vi "LED Ctlr Sys Cal Factor DPLM.vi"() -> ()   [LabVIEW 2010]
uses:
  <vilib>/Analysis/NI_AALPro.lvlib
panel:
  in  "LM Rd Dly":u32
  in  "# LEDs":u8=15
  out "Illum (Dst)":dbl format="%#_4g"
  in  "Dst Det":enum16{"Chn1", "Chn2"}(ring)=enum."Chn2"
  in  "Src Det":enum16{"Chn1", "Chn2"}(ring)
  out "error out":errorcluster
  out "Cal Factor":dbl
  out "Current Step":u16
  out "Max Illum LG":dbl caption="Gain_e" format="%.2f"
  out "Cal Factor LG":dbl caption="Gain_e" format="%.5g"
  out "Cal Factor HG":dbl caption="Gain_e" format="%.5g"
  out "Max Illum HG":dbl caption="Gain_e" format="%.2f"
  out "Calibration LG":cluster{dbl[], dbl[]}(graph)
  out "Calibration HG":cluster{dbl[], dbl[]}(graph)
  in  "OK":bool
  out "Status":string
  out "LG Dst Array":dbl[](array[numeric])
  out "HG Dst Array":dbl[](array[numeric])
  out "LG Src Array":dbl[](array[numeric])
  out "HG Src Array":dbl[](array[numeric])
  out "Inten % (Desired)":dbl
  out "Illum (Src)":dbl format="%#_4g"
  in  "DAC Higher Limit":u32=5500
  in  "DAC Lower Limit":u32=300
  in  "Number of Steps":u32=21
  in  "Wavelength":string="1550"
  in  "LED Driver Com Port":refnum<visa-resource-name>="COM9"
  in  "Light Meter Port":refnum<visa-resource-name>="COM5"
  in  "error in (no error)":errorcluster
  # "Ver 1"
  # "Cal Factor Generator (LEDAD)"
  # "ms"
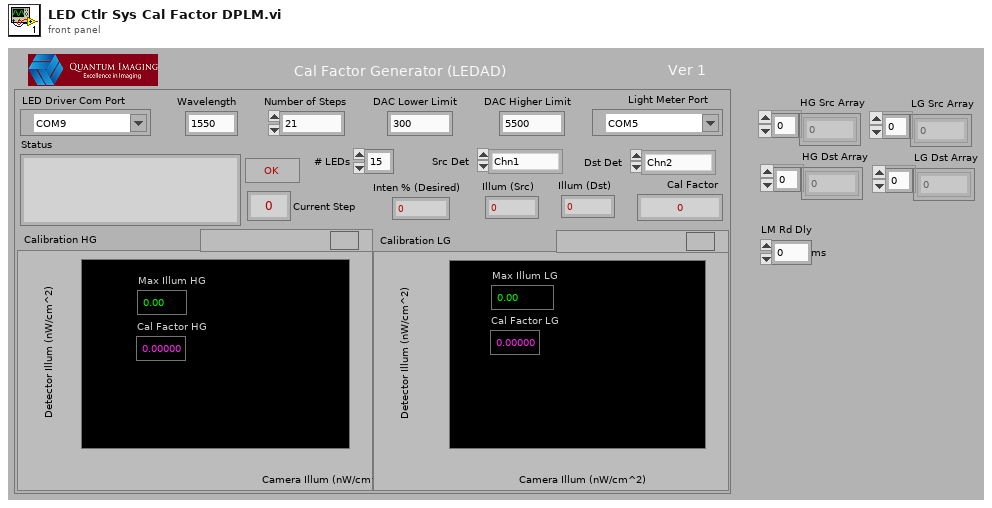
[diagram p1: front panel]
types:
  T1 = cluster{"HG Dst Array":dbl[], "HG Src Array":dbl[]}
  T2 = cluster{"LG Dst Array":dbl[], "LG Src Array":dbl[]}
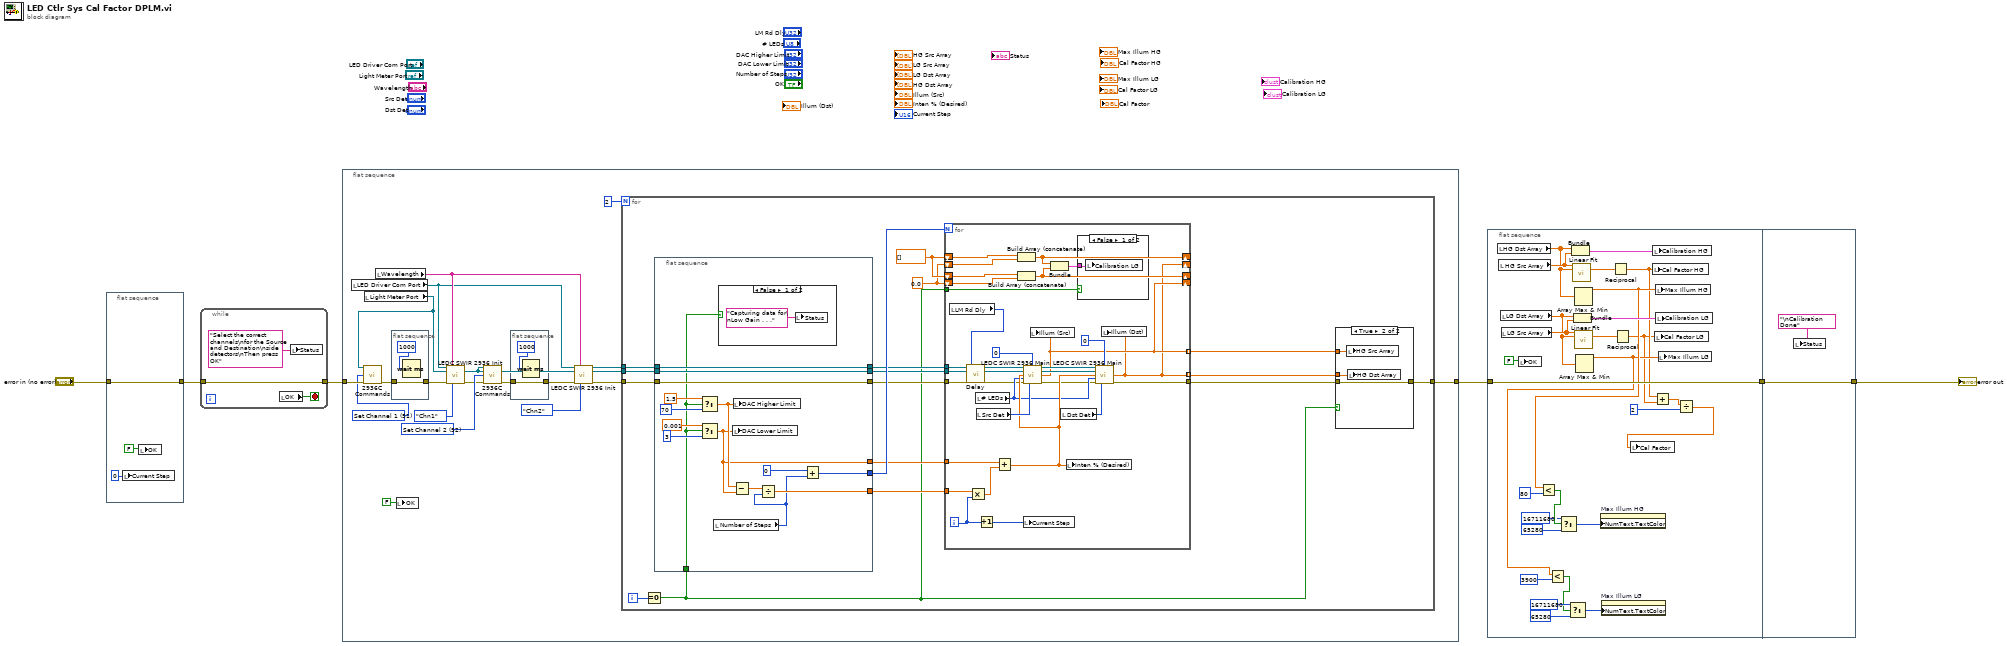
[diagram p0: block diagram]
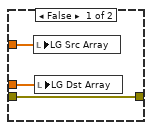
[diagram p2: hidden frame]
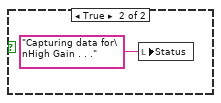
[diagram p3: hidden frame]
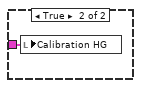
[diagram p4: hidden frame]
diagram:
  n1 = flat-sequence {
    tunnel: "error in (no error)" -> [w7]
    tunnel: [w7] -> w5
    frame #0 {
      n2 = local write "Current Step"(0) -> ()
      n3 = local write "OK"(FALSE) -> ()
    }
  }
  n4 = while {
    tunnel: [w12] -> w4
    tunnel: w5 -> [w12]
    stop <- w10 stop-if-true
    n5 = local read "OK"() -> (w10:bool)
    n6 = local write "Status"("Select the correct channels\nfor the Source and Destination\nside detectors\nThen press OK") -> ()
  }
  n7 = flat-sequence {
    tunnel: w4 -> [w25]
    tunnel: [w32] -> w3
    frame #0 {
      w18 = u16 52 items=["Attenuator OFF", "Attenuator ON", "Attenuator Query", "Beep OFF", "Beep ON", "Beep Query", "Clear Status Reg", "Get Power (nW)", "Echo OFF", "Echo ON", "Echo Query", "No Filter", "Analog Filter", "Digital FIlter", "Filter Query", "Hold", "Go", "Go Query", "Backlight OFF", "Backlight Medium", "Backlight High", "Backlight Query", "Set Dsplay Screen 0", "Set Display Screen 1", "Display Screen Query", "Mode DC Continuous", "Mode DC Single", "Mode Integrate", "Identification", "Auto Range", "Auto Range Query", "Signal Range 0", "Signal Range 1", "Signal Range 2", "Signal Range 3", "Signal Range 4", "Signal Range 5", "Signal Range 6", "Signal Range Query", "Store Reference", "Units W", "Units W/cm2", "Units dBm", "Units Joules", "Units Query", "Set Wavelength", "Wavelength Querry", "Mode Pesk-to-Peak Cont.", "Mode Peak-to-Peak Sing.", "Mode Query", "Channel Querry", "Set Channel 1", "Set Channel 2"] ("Command")
      w22 = u16 51 items=["Attenuator OFF", "Attenuator ON", "Attenuator Query", "Beep OFF", "Beep ON", "Beep Query", "Clear Status Reg", "Get Power (nW)", "Echo OFF", "Echo ON", "Echo Query", "No Filter", "Analog Filter", "Digital FIlter", "Filter Query", "Hold", "Go", "Go Query", "Backlight OFF", "Backlight Medium", "Backlight High", "Backlight Query", "Set Dsplay Screen 0", "Set Display Screen 1", "Display Screen Query", "Mode DC Continuous", "Mode DC Single", "Mode Integrate", "Identification", "Auto Range", "Auto Range Query", "Signal Range 0", "Signal Range 1", "Signal Range 2", "Signal Range 3", "Signal Range 4", "Signal Range 5", "Signal Range 6", "Signal Range Query", "Store Reference", "Units W", "Units W/cm2", "Units dBm", "Units Joules", "Units Query", "Set Wavelength", "Wavelength Querry", "Mode Pesk-to-Peak Cont.", "Mode Peak-to-Peak Sing.", "Mode Query", "Channel Querry", "Set Channel 1", "Set Channel 2"] ("Command")
      n8 = local read "LED Driver Com Port"() -> (w15:refnum<visa-resource-name>)
      n9 = local read "Light Meter Port"() -> (w23:refnum<visa-resource-name>)
      n10 = call "2936C Commands.vi"("Instrument Resource Name"=w23, "Command"=w22, "error in (no error)"=w25) -> ("error out"=w24:errorcluster)  [unwired: 8 in, 4 out]
      n11 = local read "Wavelength"() -> (w29:string)
      n12 = flat-sequence {
        tunnel: [w36] -> w20
        tunnel: w24 -> [w36]
        frame #0 {
          n13 = Wait (ms)(milliseconds to wait=1000) -> ()  [unwired: 1 out]
        }
      }
      n14 = local write "OK"(FALSE) -> ()
      n15 = call "LEDC SWIR 2936 Init.vi"("LEDAD Port"=w15, "Wavelength"=w29, "Light Meter Port"=w23, "error in (no error)"=w20, "Channel"=enum16{"Chn1", "Chn2"}."Chn1") -> ("Light Meter Port out"=w19:refnum<visa-resource-name>, "error out"=w17:errorcluster)  [unwired: 6 in, 3 out]
      n16 = call "2936C Commands.vi"("Instrument Resource Name"=w19, "Command"=w18, "error in (no error)"=w17) -> ("error out"=w13:errorcluster)  [unwired: 8 in, 4 out]
      n17 = flat-sequence {
        tunnel: [w34] -> w16
        tunnel: w13 -> [w34]
        frame #0 {
          n18 = Wait (ms)(milliseconds to wait=1000) -> ()  [unwired: 1 out]
        }
      }
      n19 = call "LEDC SWIR 2936 Init.vi"("LEDAD Port"=w15, "Wavelength"=w29, "Light Meter Port"=w19, "error in (no error)"=w16, "Channel"=enum16{"Chn1", "Chn2"}."Chn2") -> ("LEDAD Port out"=w28:refnum<visa-resource-name>, "Light Meter Port out"=w27:refnum<visa-resource-name>, "error out"=w26:errorcluster)  [unwired: 6 in, 2 out]
      n20 = for {
        N: 2 -> [_]
        tunnel: w28 -> [w48]
        tunnel: w27 -> [w47]
        tunnel: w26 -> [w46]
        tunnel: [w41] -> w32
        i -> [w52]
        w37 = 0.0
        w38 = dbl[] []
        n21 = Equal To 0?(x=w52) -> (x = 0?=w39:bool)
        n22 = flat-sequence {
          tunnel: w39 -> [w62]
          tunnel: [w67] -> w51
          tunnel: [w66] -> w50
          tunnel: [w61] -> w49
          tunnel: [w65] -> w45
          tunnel: w48 -> [w65]
          tunnel: [w64] -> w44
          tunnel: w47 -> [w64]
          tunnel: [w63] -> w43
          tunnel: w46 -> [w63]
          frame #0 {
            n23 = Select(t=1.5, s=w62, f=70) -> (s? t:f=w68:dbl)
            n24 = Select(t=0.001, s=w62, f=3) -> (s? t:f=w66:dbl)
            n25 = local read "Number of Steps"() -> (w60:u32)
            n26 = case shown="False" w62 {
              frame False {
                n27 = local write "Status"("Capturing data for\nLow Gain . . .") -> ()
              }
              frame True {
                n28 = local write "Status"("Capturing data for\nHigh Gain . . .") -> ()
              }
            }
            n29 = local write "DAC Lower Limit"(w66) -> ()
            n30 = local write "DAC Higher Limit"(w68) -> ()
            n31 = Subtract(x=w68, y=w66) -> (x-y=w73:dbl)
            n32 = Divide(x=w73, y=w60) -> (x/y=w61:dbl)
            n33 = Add(x=0, y=w60) -> (x+y=w67:u32)
          }
        }
        n34 = for {
          N: w51 -> [_]
          tunnel: w45 -> [w106]
          tunnel: w44 -> [w105]
          tunnel: w43 -> [w79]
          tunnel: w49 -> [w103]
          tunnel: w50 -> [w101]
          tunnel: [w84] -> w53 mode=indexing
          tunnel: [w81] -> w42
          tunnel: [w83] -> w40 mode=indexing
          shift-right: [w92] -> _
          shift-left: w38 -> [w91]
          shift-right: [w83] -> _
          shift-left: w37 -> [w90]
          shift-right: [w87] -> _
          shift-left: w38 -> [w89]
          shift-right: [w84] -> _
          shift-left: w37 -> [w88]
          tunnel: w39 -> [w86]
          i -> [w100]
          n35 = local read "LM Rd Dly"() -> (w77:u32)
          n36 = call "Delay.vi"("error in (no error)"=w79, "Delay"=w77) -> ("error out"=w78:errorcluster)  [unwired: 17 in]
          n37 = Multiply(x=w103, y=w100) -> (x*y=w102:dbl)
          n38 = local read "# LEDs"() -> (w82:u8)
          n39 = local read "Src Det"() -> (w94:enum16{"Chn1", "Chn2"})
          n40 = Increment(x=w100) -> (x+1=w99:i32)
          n41 = Add(x=w101, y=w102) -> (x+y=w93:dbl)
          n42 = Build Array (concatenate)(w91, w90) -> (w92:dbl[])
          n43 = Build Array (concatenate)(w89, w88) -> (w87:dbl[])
          n44 = call "LEDC SWIR 2936 Main.vi"("LEDAD Port"=w106, "Unit"=0, "Light Meter Port"=w105, "Intensity Desired"=w93, "Enable LED"=w82, "error in (no error)"=w78, "Channel"=w94) -> ("LEDAD Port out"=w97:refnum<visa-resource-name>, "Light Meter Port out"=w96:refnum<visa-resource-name>, "Meas Illum"=w84:dbl, "error out"=w80:errorcluster)  [unwired: 3 in, 2 out]
          n45 = local write "Current Step"(w99) -> ()
          n46 = local write "Illum (Src)"(w84) -> ()
          n47 = Bundle(w92, w87) -> (w85:cluster{dbl[], dbl[]})  [unwired: 1 in]
          n48 = local read "Dst Det"() -> (w95:enum16{"Chn1", "Chn2"})
          n49 = local write "Inten % (Desired)"(w93) -> ()
          n50 = case shown="False" w86 {
            tunnel: w85 -> [w107 w108]
            frame False {
              n51 = local write "Calibration LG"(w107) -> ()
            }
            frame True {
              n52 = local write "Calibration HG"(w108) -> ()
            }
          }
          n53 = call "LEDC SWIR 2936 Main.vi"("LEDAD Port"=w97, "Unit"=0, "Light Meter Port"=w96, "Intensity Desired"=w93, "Enable LED"=w82, "error in (no error)"=w80, "Channel"=w95) -> ("Meas Illum"=w83:dbl, "error out"=w81:errorcluster)  [unwired: 3 in, 4 out]
          n54 = local write "Illum (Dst)"(w83) -> ()
        }
        n55 = case shown="True" w39 {
          tunnel: w53 -> [w56 w59]
          tunnel: [w55 w58] -> w41
          tunnel: w42 -> [w55 w58]
          tunnel: w40 -> [w54 w57]
          frame False {
            n56 = local write "LG Src Array"(w56) -> ()
            n57 = local write "LG Dst Array"(w54) -> ()
          }
          frame True {
            n58 = local write "HG Src Array"(w59) -> ()
            n59 = local write "HG Dst Array"(w57) -> ()
          }
        }
      }
    }
  }
  n60 = flat-sequence {
    tunnel: w3 -> [w129]
    tunnel: [w129] -> w1
    tunnel: [w137] -> w2
    tunnel: w1 -> [w137]
    frame #0 {
      n61 = local read "HG Dst Array"() -> (w127:dbl[])
      n62 = local read "HG Src Array"() -> (w135:dbl[])
      n63 = local read "LG Dst Array"() -> (w126:dbl[])
      n64 = local read "LG Src Array"() -> (w132:dbl[])
      n65 = local write "OK"(FALSE) -> ()
      n66 = Bundle("HG Dst Array"=w127, "HG Src Array"=w135) -> (w134:T1)  [unwired: 1 in]
      n67 = call <vilib>:"Linear Fit.vi"("Y"=w135, "X"=w127) -> ("slope"=w112:dbl)  [unwired: 9 in, 4 out]
      n68 = Bundle("LG Dst Array"=w126, "LG Src Array"=w132) -> (w133:T2)  [unwired: 1 in]
      n69 = Array Max & Min(array=w127) -> (max value=w115:dbl)  [unwired: 3 out]
      n70 = Less?(x=w115, y=80) -> (x < y?=w125:bool)
      n71 = Select(t=u32 16711680, s=w125, f=u32 65280) -> (s? t:f=w121:u32)
      n72 = call <vilib>:"Linear Fit.vi"("Y"=w132, "X"=w126) -> ("slope"=w110:dbl)  [unwired: 9 in, 4 out]
      n73 = Array Max & Min(array=w126) -> (max value=w114:dbl)  [unwired: 3 out]
      n74 = Less?(x=w114, y=3900) -> (x < y?=w117:bool)
      n75 = Select(t=u32 16711680, s=w117, f=u32 65280) -> (s? t:f=w116:u32)
      n76 = property on="Max Illum HG" class="DigNum (strict)"("NumText.TextColor"=w121) -> ()  [unwired: 2 in, 2 out]
      n77 = property on="Max Illum LG" class="DigNum (strict)"("NumText.TextColor"=w116) -> ()  [unwired: 2 in, 2 out]
      n78 = Reciprocal(x=w112) -> (1/x=w111:dbl)
      n79 = Reciprocal(x=w110) -> (1/x=w109:dbl)
      n80 = local write "Cal Factor HG"(w111) -> ()
      n81 = local write "Calibration HG"(w134) -> ()
      n82 = Add(x=w111, y=w109) -> (x+y=w130:dbl)
      n83 = local write "Cal Factor LG"(w109) -> ()
      n84 = local write "Max Illum HG"(w115) -> ()
      n85 = local write "Calibration LG"(w133) -> ()
      n86 = local write "Max Illum LG"(w114) -> ()
      n87 = Divide(x=w130, y=2) -> (x/y=w128:dbl)
      n88 = local write "Cal Factor"(w128) -> ()
    }
    frame #1 {
      n89 = local write "Status"("\nCalibration Done") -> ()
    }
  }
  "error out" <- w2
